vi "水质测量数据table定义.vi"(5 "数据标记表":string(combo)="N", 7 "table 输入":string, 9 "SN":string, 10 "测量模式":T1(ring)=enum."水样测试", 11 "data":T3 {"单位" items=["ug/L", "mg/L", "ppm", "mg/m3", "cm", "ppb", "ug/m3", "%", "nmol/mol", "umol/mol", "MPN/L", "MPN/100ml", "ng/m3", "NTU", "无量纲", "ms/cm", "us/cm"]}) -> (1 "table 输出":string, 2 "columns":string[](array[string]), 3 "data输出":T2)   [LabVIEW 2016, in "database.lvlib"]
uses:
  database.lvlib
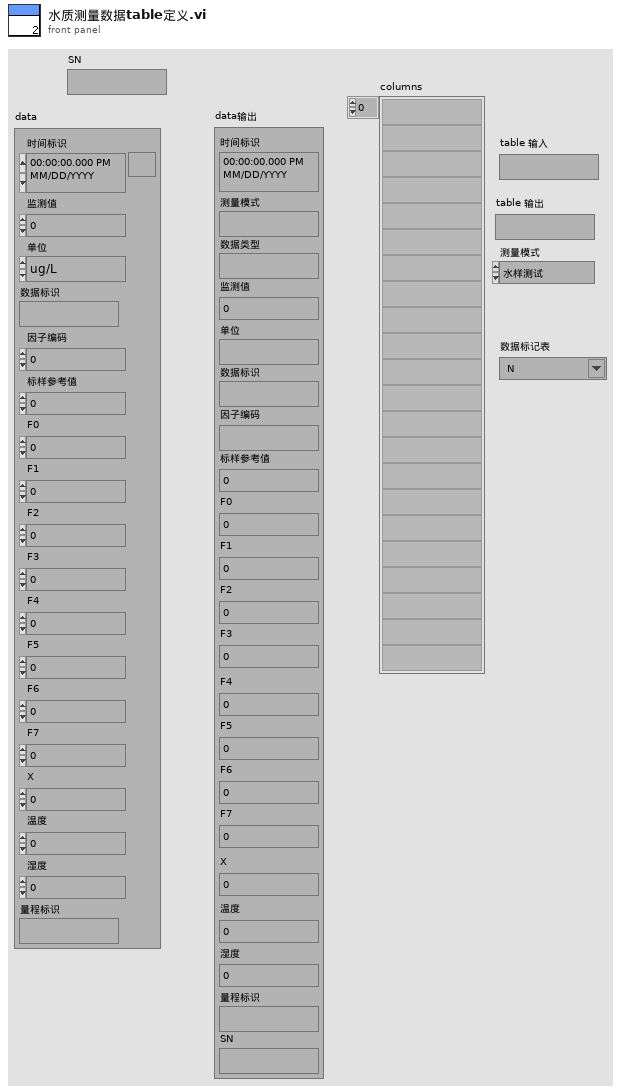
[diagram p1: front panel]
types:
  T1 = enum16{"维护数据", "水样测试", "标样核查", "零点核查", "跨度核查", "空白测试", "平行样测试", "加标回收", "空白校准", "标样校准", "初始化（清洗）"}
  T2 = cluster{"时间标识":timestamp, "测量模式":string, "数据类型":string, "监测值":sgl, "单位":string, "数据标识":string, "因子编码":string, "标样参考值":sgl, "F0":sgl, "F1":sgl, "F2":sgl, "F3":sgl, "F4":sgl, "F5":sgl, "F6":sgl, "F7":sgl, "X":sgl, "温度":sgl, "湿度":sgl, "量程标识":string, "SN":string}
  T3 = cluster{"时间标识":timestamp, "监测值":sgl, "单位":u16, "数据标识":string, "因子编码":u32, "标样参考值":sgl, "F0":sgl, "F1":sgl, "F2":sgl, "F3":sgl, "F4":sgl, "F5":sgl, "F6":sgl, "F7":sgl, "X":sgl, "温度":sgl, "湿度":sgl, "量程标识":string}
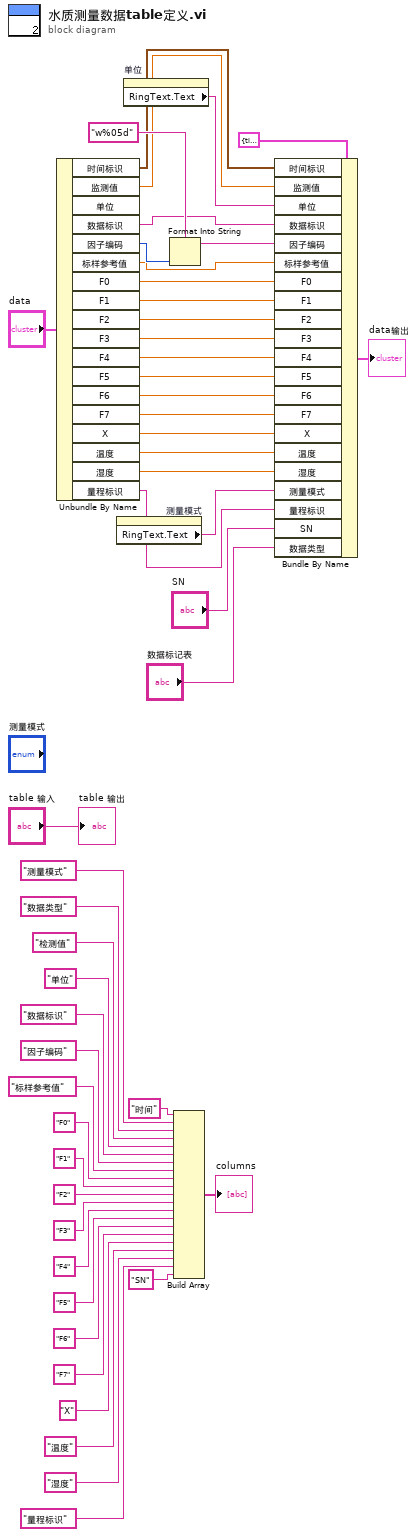
[diagram p0: block diagram]
diagram:
  n1 = Unbundle By Name("data") -> ("时间标识"=w33:timestamp, "监测值"=w32:sgl, "数据标识"=w31:string, "因子编码"=w37:u32, "标样参考值"=w22:sgl, "F0"=w23:sgl, "F1"=w30:sgl, "F2"=w29:sgl, "F3"=w28:sgl, "F4"=w10:sgl, "F5"=w9:sgl, "F6"=w8:sgl, "F7"=w7:sgl, "X"=w6:sgl, "温度"=w27:sgl, "湿度"=w26:sgl, "量程标识"=w17:string)  [unwired: 1 out]
  n2 = property on="测量模式" class="Enum (strict)"() -> ("RingText.Text"=w19:string)  [unwired: 2 in, 2 out]
  n3 = property on="单位" class="Ring (strict)"() -> ("RingText.Text"=w25:string)  [unwired: 2 in, 2 out]
  n4 = Format Into String(format string="w%05d" ("格式字符串"), w37) -> (resulting string=w34:string)  [unwired: 2 in, 1 out]
  n5 = Build Array("时间", "测量模式", "数据类型", "检测值", "单位", "数据标识", "因子编码", "标样参考值", "F0", "F1", "F2", "F3", "F4", "F5", "F6", "F7", "X", "温度", "湿度", "量程标识", "SN") -> (→"columns":string[])
  n6 = Bundle By Name(cluster=T2 {"时间标识"=timestamp(0 s since 1904-01-01), "测量模式"="", "数据类型"="", "监测值"=0.0, "单位"="", "数据标识"="", "因子编码"="", "标样参考值"=0.0, "F0"=0.0, "F1"=0.0, "F2"=0.0, "F3"=0.0, "F4"=0.0, "F5"=0.0, "F6"=0.0, "F7"=0.0, "X"=0.0, "温度"=0.0, "湿度"=0.0, "量程标识"="", "SN"=""} ("data输出"), "时间标识"=w33, "监测值"=w32, "单位"=w25, "数据标识"=w31, "因子编码"=w34, "标样参考值"=w22, "F0"=w23, "F1"=w30, "F2"=w29, "F3"=w28, "F4"=w10, "F5"=w9, "F6"=w8, "F7"=w7, "X"=w6, "温度"=w27, "湿度"=w26, "测量模式"=w19, "量程标识"=w17, "SN"="SN", "数据类型"="数据标记表") -> (→"data输出":T2)
  "table 输出" <- "table 输入"
